vi "AO_v2_4x1darray.vi"() -> ()   [LabVIEW 2023]
panel:
  out "Loop Execution Time":u32
  out "size(s) 8":i32
  out "size(s) 7":i32
  out "Time":dbl[](array[numeric])
  out "size(s) 6":i32
  out "size(s) 5":i32
  out "Density":dbl[](array[numeric])
  out "size(s) 4":i32
  out "size(s) 3":i32
  out "Temperature":dbl[](array[numeric])
  out "size(s) 2":i32
  out "size(s)":i32
  out "Pressure":dbl[](array[numeric])
  out "current time":timestamp
  out "startr_time":timestamp
  out "Waveform Chart":waveform(dbl)(graph)
  in  "Number of Samples":i32=1000
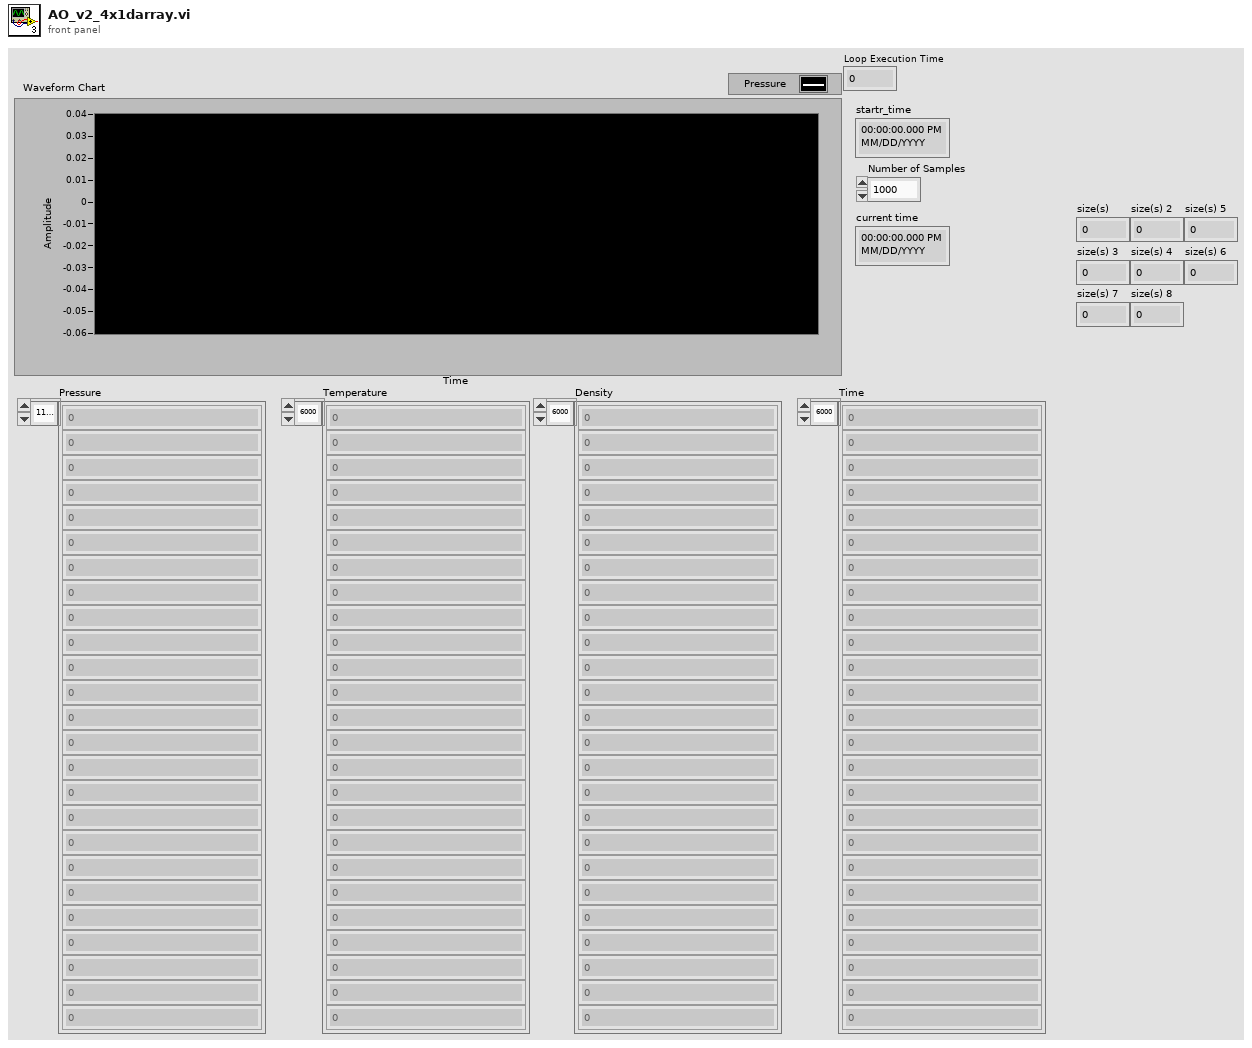
[diagram p1: front panel]
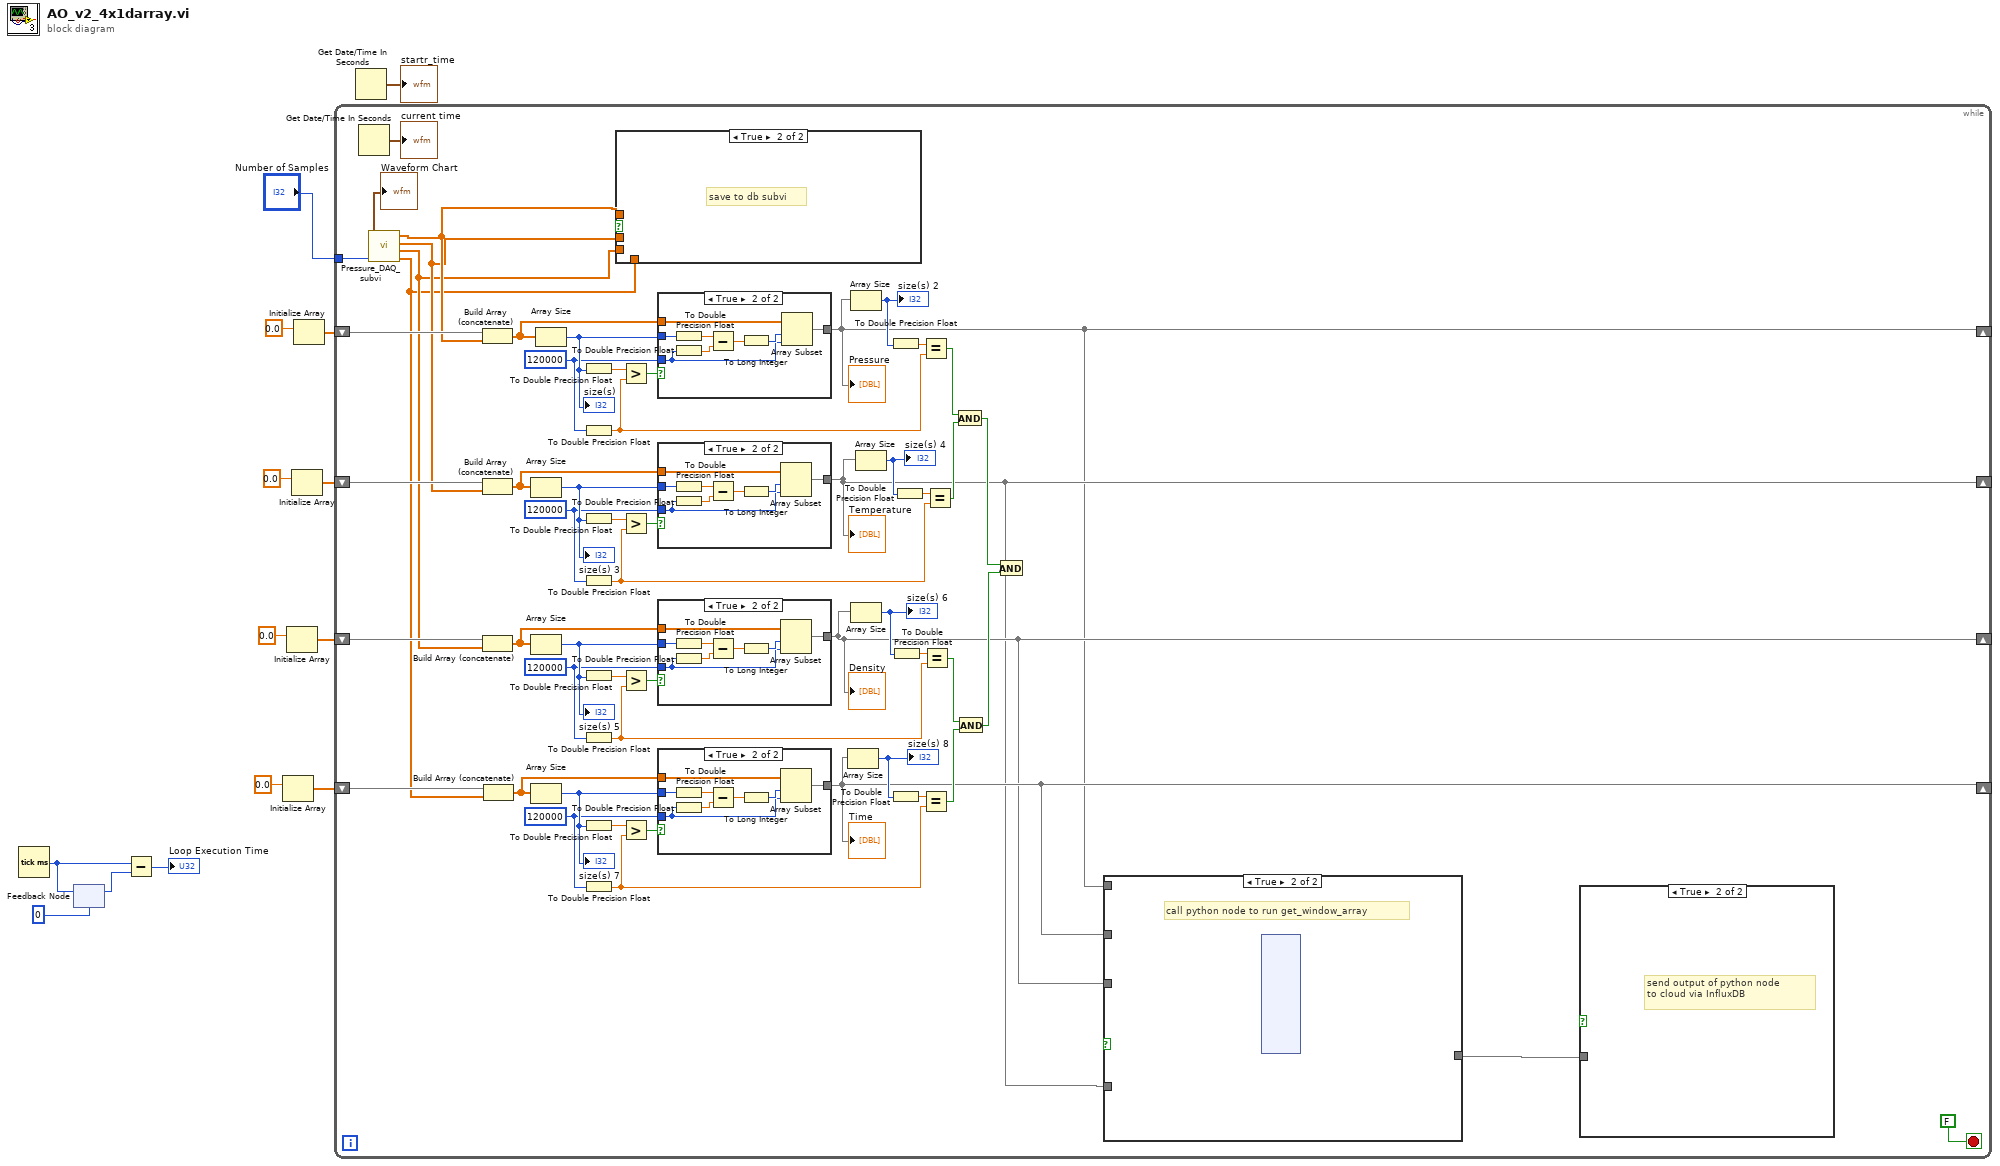
[diagram p0: block diagram]
diagram:
  n1 = Tick Count (ms)() -> (millisecond timer value=w2:u32)
  n2 = feedback #1(u32 0) -> (w3:u32)
  n3 = feedback-in #1(w2) -> ()
  n4 = Subtract(x=w2, y=w3) -> (x-y=→"Loop Execution Time":u32)
  n5 = Initialize Array(0.0 ("element")) -> (w6:dbl[])  [unwired: 1 in]
  n6 = Initialize Array(0.0 ("element")) -> (w5:dbl[])  [unwired: 1 in]
  n7 = Initialize Array(0.0 ("element")) -> (w9:dbl[])  [unwired: 1 in]
  n8 = Initialize Array(0.0 ("element")) -> (w12:dbl[])  [unwired: 1 in]
  n9 = while {
    tunnel: "Number of Samples" -> [w66]
    shift-right: [w16] -> _
    shift-left: w12 -> [w65]
    shift-right: [w17] -> _
    shift-left: w9 -> [w44]
    shift-right: [w18] -> _
    shift-left: w5 -> [w42]
    shift-right: [w19] -> _
    shift-left: w6 -> [w43]
    stop <- FALSE stop-if-true
    w45 = 120000
    w50 = 120000
    w55 = 120000
    w60 = 120000
    n10 = Get Date/Time In Seconds() -> (seconds since 1Jan1904=→"current time":timestamp)
    n11 = call "Pressure_DAQ_subvi.vi"("Number of Samples"=w66) -> ("Waveform Chart"=→"Waveform Chart":waveform(dbl), "pressure_Vdc"=w23:dbl[], "density_constant"=w22:dbl[], "temp_constant"=w21:dbl[], "unix_time"=w20:dbl[])  [unwired: 5 in]
    n12 = Build Array (concatenate)(w65, w23) -> (w64:dbl[])
    n13 = Build Array (concatenate)(w44, w22) -> (w59:dbl[])
    n14 = Build Array (concatenate)(w42, w21) -> (w54:dbl[])
    n15 = Build Array (concatenate)(w43, w20) -> (w49:dbl[])
    n16 = Array Size(array=w59) -> (size(s)=w56:i32)
    "size(s) 3" <- w56
    n17 = Array Size(array=w54) -> (size(s)=w51:i32)
    "size(s) 5" <- w51
    n18 = Array Size(array=w49) -> (size(s)=w46:i32)
    "size(s) 7" <- w46
    n19 = Array Size(array=w64) -> (size(s)=w61:i32)
    "size(s)" <- w61
    n20 = To Double Precision Float(number=w61) -> (double precision float=w63:dbl)
    n21 = To Double Precision Float(number=w60) -> (double precision float=w39:dbl)
    n22 = To Double Precision Float(number=w56) -> (double precision float=w58:dbl)
    n23 = To Double Precision Float(number=w55) -> (double precision float=w36:dbl)
    n24 = To Double Precision Float(number=w51) -> (double precision float=w53:dbl)
    n25 = To Double Precision Float(number=w50) -> (double precision float=w27:dbl)
    n26 = To Double Precision Float(number=w46) -> (double precision float=w48:dbl)
    n27 = To Double Precision Float(number=w45) -> (double precision float=w26:dbl)
    n28 = case shown="True" {
      selector: _ -> [_ _]
      tunnel: [_ w70] -> _
      tunnel: w23 -> [_ w70]
      tunnel: w22 -> [_ _]
      tunnel: w21 -> [_ _]
      tunnel: w20 -> [_ _]
      frame False {
      }
      frame True {
        # "save to db subvi"
      }
    }
    n29 = Greater?(x=w63, y=w39) -> (0:w62:bool)
    n30 = Greater?(x=w58, y=w36) -> (0:w57:bool)
    n31 = Greater?(x=w53, y=w27) -> (0:w52:bool)
    n32 = Greater?(x=w48, y=w26) -> (0:w47:bool)
    n33 = case shown="True" w62 {
      tunnel: [w98 w106] -> w16
      tunnel: w64 -> [w98 w105]
      tunnel: w61 -> [_ w101]
      tunnel: w60 -> [_ w99]
      frame False {
      }
      frame True {
        n34 = To Double Precision Float(number=w101) -> (double precision float=w104:dbl)
        n35 = To Double Precision Float(number=w99) -> (double precision float=w103:dbl)
        n36 = Subtract(x=w104, y=w103) -> (x-y=w102:dbl)
        n37 = To Long Integer(number=w102) -> (32bit integer=w100:i32)
        n38 = Array Subset(array=w105, index=w100, length=w99) -> (w106:dbl[])
      }
    }
    "Pressure" <- w16
    n39 = case shown="True" w57 {
      tunnel: [w89 w97] -> w17
      tunnel: w59 -> [w89 w96]
      tunnel: w56 -> [_ w92]
      tunnel: w55 -> [_ w90]
      frame False {
      }
      frame True {
        n40 = To Double Precision Float(number=w92) -> (double precision float=w95:dbl)
        n41 = To Double Precision Float(number=w90) -> (double precision float=w94:dbl)
        n42 = Subtract(x=w95, y=w94) -> (x-y=w93:dbl)
        n43 = To Long Integer(number=w93) -> (32bit integer=w91:i32)
        n44 = Array Subset(array=w96, index=w91, length=w90) -> (w97:dbl[])
      }
    }
    "Temperature" <- w17
    n45 = case shown="True" w52 {
      tunnel: [w80 w88] -> w18
      tunnel: w54 -> [w80 w87]
      tunnel: w51 -> [_ w83]
      tunnel: w50 -> [_ w81]
      frame False {
      }
      frame True {
        n46 = To Double Precision Float(number=w83) -> (double precision float=w86:dbl)
        n47 = To Double Precision Float(number=w81) -> (double precision float=w85:dbl)
        n48 = Subtract(x=w86, y=w85) -> (x-y=w84:dbl)
        n49 = To Long Integer(number=w84) -> (32bit integer=w82:i32)
        n50 = Array Subset(array=w87, index=w82, length=w81) -> (w88:dbl[])
      }
    }
    "Density" <- w18
    n51 = case shown="True" w47 {
      tunnel: [w71 w79] -> w19
      tunnel: w49 -> [w71 w78]
      tunnel: w46 -> [_ w74]
      tunnel: w45 -> [_ w72]
      frame False {
      }
      frame True {
        n52 = To Double Precision Float(number=w74) -> (double precision float=w77:dbl)
        n53 = To Double Precision Float(number=w72) -> (double precision float=w76:dbl)
        n54 = Subtract(x=w77, y=w76) -> (x-y=w75:dbl)
        n55 = To Long Integer(number=w75) -> (32bit integer=w73:i32)
        n56 = Array Subset(array=w78, index=w73, length=w72) -> (w79:dbl[])
      }
    }
    "Time" <- w19
    n57 = Array Size(array=w19) -> (size(s)=w32:i32)
    "size(s) 8" <- w32
    n58 = Array Size(array=w16) -> (size(s)=w40:i32)
    "size(s) 2" <- w40
    n59 = Array Size(array=w18) -> (size(s)=w33:i32)
    "size(s) 6" <- w33
    n60 = Array Size(array=w17) -> (size(s)=w37:i32)
    "size(s) 4" <- w37
    n61 = To Double Precision Float(number=w40) -> (double precision float=w41:dbl)
    n62 = To Double Precision Float(number=w32) -> (double precision float=w34:dbl)
    n63 = To Double Precision Float(number=w33) -> (double precision float=w35:dbl)
    n64 = To Double Precision Float(number=w37) -> (double precision float=w38:dbl)
    n65 = Equal?(x=w41, y=w39) -> (x = y?=w31:bool)
    n66 = Equal?(x=w34, y=w26) -> (x = y?=w28:bool)
    n67 = Equal?(x=w35, y=w27) -> (x = y?=w29:bool)
    n68 = Equal?(x=w38, y=w36) -> (x = y?=w30:bool)
    n69 = And(x=w31, y=w30) -> (x .and. y?=w24:bool)
    n70 = And(x=w29, y=w28) -> (x .and. y?=w25:bool)
    n71 = And(x=w24, y=w25) -> ()  [unwired: 1 out]
    n72 = case shown="True" {
      selector: _ -> [_ _]
      tunnel: [_ _] -> w15
      frame False {
      }
      frame True {
        # "send output of python node \nto cloud via InfluxDB"
      }
    }
    n73 = case shown="True" {
      selector: _ -> [_ _]
      tunnel: w19 -> [_ _]
      tunnel: w18 -> [_ _]
      tunnel: w17 -> [_ _]
      tunnel: w16 -> [_ _]
      tunnel: w15 -> [_ _]
      frame False {
      }
      frame True {
        # "call python node to run get_window_array"
        n74 = node() -> ()  [unwired: 26 in, 4 out]
      }
    }
  }
  n75 = Get Date/Time In Seconds() -> (seconds since 1Jan1904=→"startr_time":timestamp)
